vi "SubVI_ShrinkArray_001.vi"(1 "Input Array":i32[](array[numeric])) -> (0 "Output Array":i32[](array[numeric]))   [LabVIEW 2018]
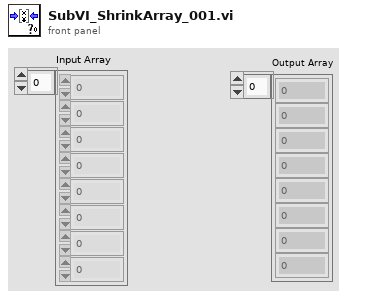
[diagram p1: front panel]
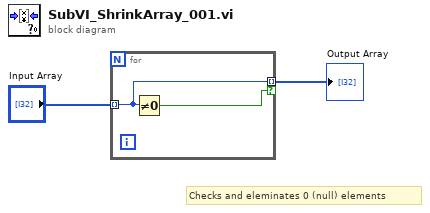
[diagram p0: block diagram]
diagram:
  # "Checks and eleminates 0 (null) elements"
  n1 = for {
    tunnel: "Input Array" -> [w4] mode=indexing
    tunnel: [w4] -> w1 mode=indexing if=w3
    n2 = Not Equal To 0?(x=w4) -> (x != 0?=w3:bool)
  }
  "Output Array" <- w1
